vi "combining_waveforms.vi"() -> ()   [LabVIEW 2023]
uses:
  <vilib>/Analysis/3filter.llb/Filter Passband Type.ctl
  <vilib>/Analysis/3filter.llb/Butterworth Filter (DBL).vi
  <vilib>/express/express analysis/Spectral/Block/exnSpectralBlock spectral measurements RMS poly.vi
  <vilib>/express/express analysis/Spectral/Block/exnSpectralBlock spectral measurements RMS WFM.vi
  <vilib>/express/express analysis/Spectral/XNode/ExpressSpectralMeasurementsBlockNode.xnode
  <vilib>/Analysis/NI_AALBase.lvlib
panel:
  in  "OK Button":bool
  in  "Play Sound":bool
  in  "stop":bool
  in  "Parameters":T1(array[cluster]) {"Signal" items=["Sine", "Square", "Triangle", "Sawtooth"]; "Amplitude" scale=0.0..10.0; "Frequency" scale=0.0..1000.0}
  in  "?":T3={"filter type"=enum."Lowpass", "low cutoff freq"=0.12500000000000006, "high cutoff freq"=0.45000000000000007} {"high cutoff freq" format="%0.2f"; "low cutoff freq" format="%0.4f"}
  in  "Filter OFF   Filter ON":bool
  out "Waveform Graph 2":cluster{"f0":dbl, "df":dbl, "magnitude":dbl[]}(graph)
  out "Waveform Graph":waveform(dbl)(graph)
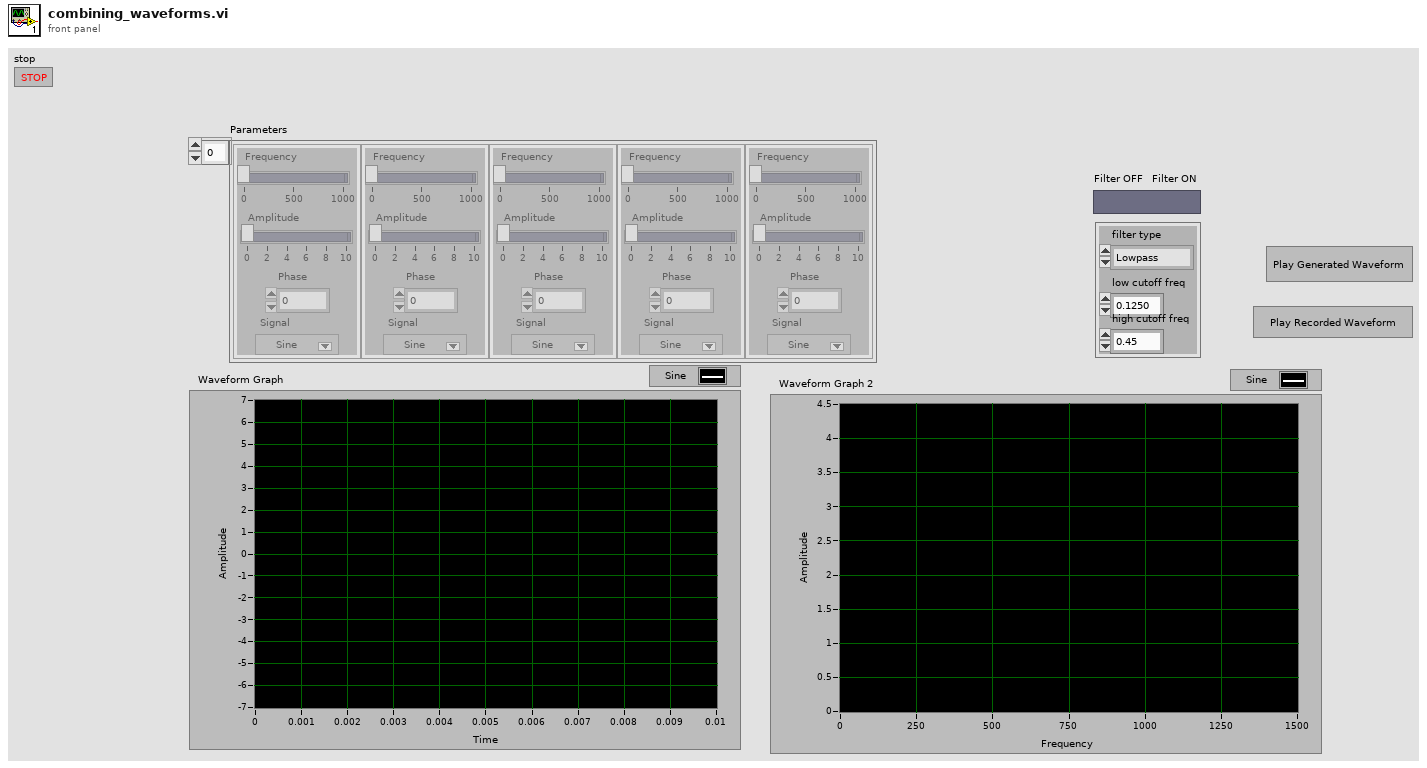
[diagram p1: front panel]
types:
  T1 = cluster{"Frequency":dbl, "Amplitude":dbl, "Signal":u16, "Phase":dbl}[]
  T2 = typedef "NI_AALBase.lvlib/Filter Passband Type.ctl" = enum32{"Lowpass", "Highpass", "Bandpass", "Bandstop"}
  T3 = cluster{"filter type":T2, "low cutoff freq":dbl, "high cutoff freq":dbl}
  T4 = cluster{"averaging mode":u16, "weighting mode":u16, "number of averages":u32}
  T5 = cluster{"dB On (F)":bool, "unwrap phase (F)":bool, "convert to degree (F)":bool}
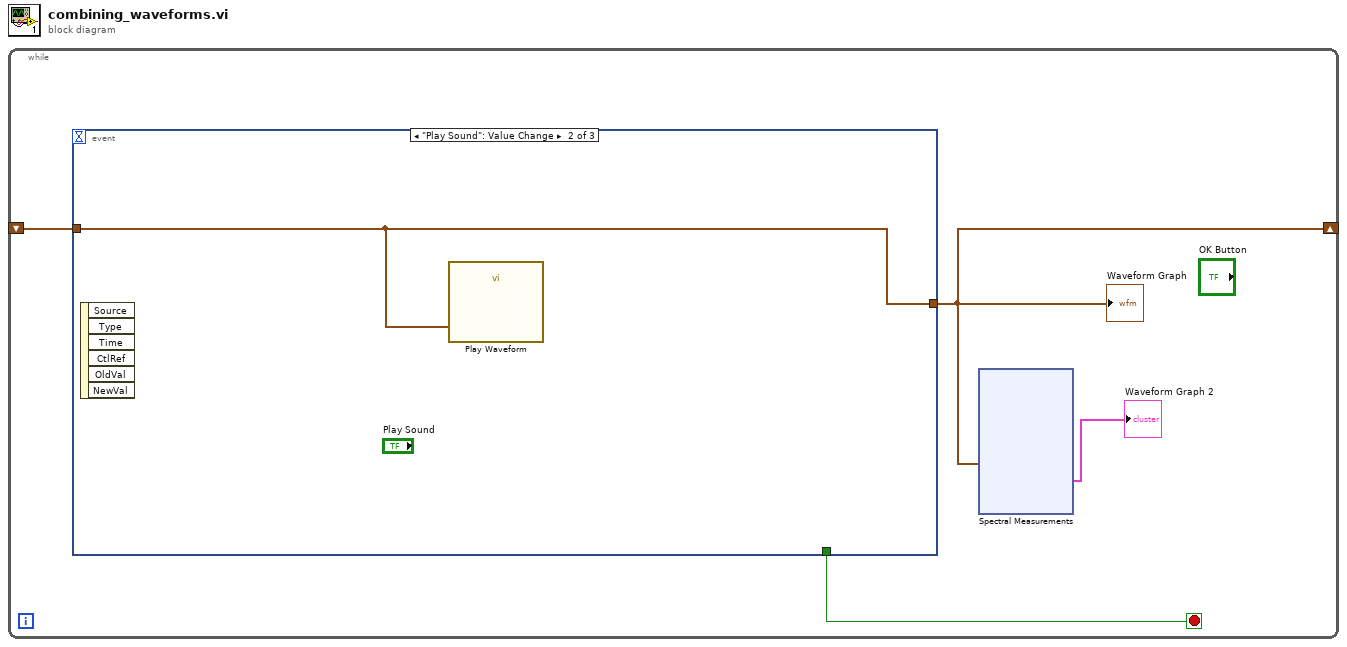
[diagram p0: block diagram]
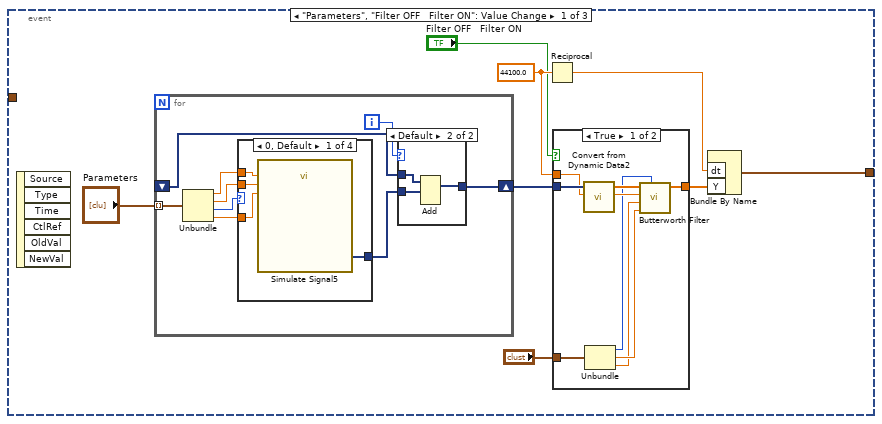
[diagram p2: hidden frame]
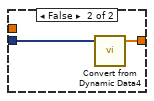
[diagram p3: hidden frame]
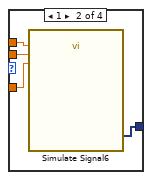
[diagram p4: hidden frame]
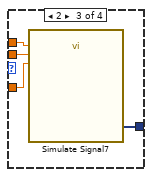
[diagram p5: hidden frame]
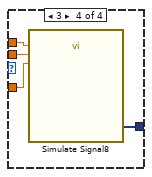
[diagram p6: hidden frame]
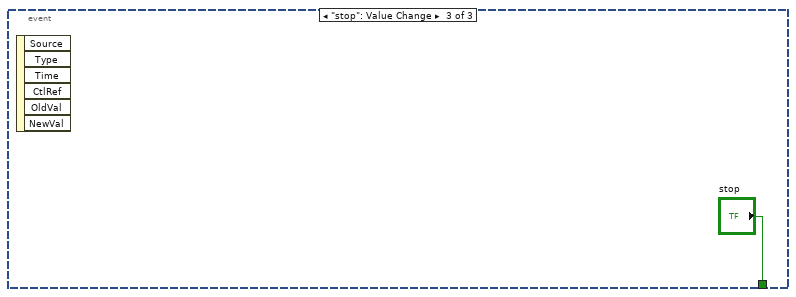
[diagram p8: hidden frame]
diagram:
  n1 = while {
    shift-right: [w1] -> _
    shift-left: _ -> [w3]
    stop <- w4 stop-if-true
    n2 = event shown="[1] \"Play Sound\": Value Change" {
      selector: _ -> [_ _ _]
      dyn-events: _ -> [_ _ _]
      timeout: _ -> [_ _ _]
      tunnel: [w15 w62 _] -> w1
      tunnel: [_ _ "stop"] -> w4
      tunnel: w3 -> [_ w62 _]
      event "Parameters", "Filter OFF   Filter ON": Value Change {
        w20 = 44100.0
        n3 = event-data() -> ()  [unwired: 1 in, 6 out]
        n4 = for {
          shift-right: [w40] -> w21
          shift-left: _ -> [w39]
          tunnel: "Parameters" -> [w38] mode=indexing
          i -> [w41]
          n5 = Unbundle(w38) -> ("Frequency"=w36:dbl, "Amplitude"=w37:dbl, "Signal"=w35:u16, "Phase"=w33:dbl)
          n6 = case shown="0, Default" w35 {
            tunnel: [w45 w49 w53 w57] -> w34
            tunnel: w37 -> [w44 w48 w52 w56]
            tunnel: w36 -> [w43 w47 w51 w55]
            tunnel: w33 -> [w42 w46 w50 w54]
            frame 0, Default {
              n7 = call "Simulate Signal5"("Frequency"=w43, "Amplitude"=w44, "Phase"=w42) -> ("Sine"=w45:dynamicdata)  [unwired: 11 in, 1 out]
            }
            frame 1 {
              n8 = call "Simulate Signal6"("Frequency"=w47, "Amplitude"=w48, "Phase"=w46) -> ("Square"=w49:dynamicdata)  [unwired: 11 in, 1 out]
            }
            frame 2 {
              n9 = call "Simulate Signal7"("Frequency"=w51, "Amplitude"=w52, "Phase"=w50) -> ("Triangle"=w53:dynamicdata)  [unwired: 11 in, 1 out]
            }
            frame 3 {
              n10 = call "Simulate Signal8"("Frequency"=w55, "Amplitude"=w56, "Phase"=w54) -> ("Sawtooth"=w57:dynamicdata)  [unwired: 11 in, 1 out]
            }
          }
          n11 = case shown="Default" w41 {
            tunnel: w34 -> [w58 w61]
            tunnel: [w58 w60] -> w40
            tunnel: w39 -> [_ w59]
            frame 0 {
            }
            frame Default {
              n12 = Add(1:w61, 2:w59) -> (0:w60:dynamicdata)  [unwired: 1 in, 1 out]
            }
          }
        }
        n13 = Reciprocal(x=w20) -> (1/x=w17:dbl)
        n14 = case shown="True" "Filter OFF   Filter ON" {
          tunnel: w21 -> [w30 w32]
          tunnel: [w28 w31] -> w16
          tunnel: w20 -> [w27 _]
          tunnel: "?" -> [w26 _]
          frame True {
            n15 = call "Convert from Dynamic Data2"("Dynamic Data Type"=w30) -> ("Array"=w29:dbl[])  [unwired: 3 in]
            n16 = Unbundle(w26) -> ("filter type"=w25:T2, "low cutoff freq"=w24:dbl, "high cutoff freq"=w23:dbl)
            n17 = call-poly <vilib>:"Butterworth Filter.vi"("filter type"=w25, "low cutoff freq: fl"=w24, "high cutoff freq: fh"=w23, "sampling freq: fs"=w27, "X"=w29) -> ("Filtered X"=w28:dbl[])  [unwired: 3 in, 1 out]
          }
          frame False {
            n18 = call "Convert from Dynamic Data4"("Dynamic Data Type"=w32) -> ("Array"=w31:dbl[])  [unwired: 3 in]
          }
        }
        n19 = Bundle By Name("dt"=w17, "Y"=w16) -> (w15:waveform(dbl))  [unwired: 1 in]
      }
      event "Play Sound": Value Change {
        n20 = event-data() -> ()  [unwired: 1 in, 6 out]
        n21 = call "Play Waveform"("Data"=w62) -> ()  [unwired: 18 in, 1 out]
      }
      event "stop": Value Change {
        n22 = event-data() -> ()  [unwired: 1 in, 6 out]
      }
    }
    "Waveform Graph" <- w1
    n23 = xnode "Spectral Measurements"("Signals"=w1) -> ("FFT - (RMS)"=→"Waveform Graph 2":cluster{"f0":dbl, "df":dbl, "magnitude":dbl[]})  [unwired: 1 in, 2 out]
  }
